vi "gwyscan create path random.vi"(5 "yoffset":dbl, 6 "xoffset":dbl, 7 "yreal":dbl, 8 "error in (no error)":errorcluster, 9 "xreal":dbl, 10 "n":i32, 11 "xypos":dbl[](array[numeric])) -> (0 "error out":errorcluster, 2 "function return":i32, 3 "xypos":dbl[](array[numeric]))   [LabVIEW 2016, in "libgwyscan.lvlib"]
doc: "GWYSCANDLL_API int gwyscan_create_path_random(double *xypos, int n, double xreal, double yreal, double xoffset, double yoffset);"
uses:
  libgwyscan.lvlib
  libgwyscan.dll
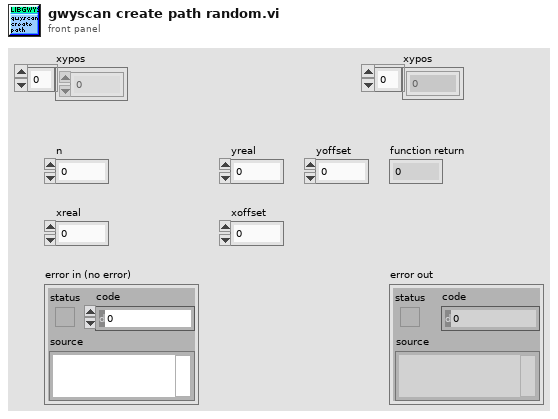
[diagram p1: front panel]
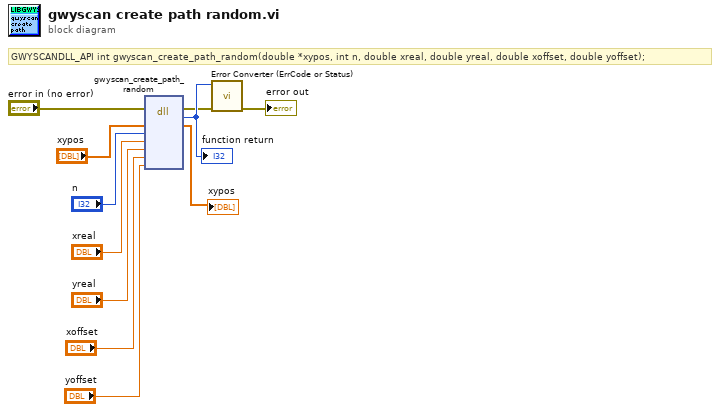
[diagram p0: block diagram]
diagram:
  # "GWYSCANDLL_API int gwyscan_create_path_random(double *xypos, int n, double xreal, double yreal, double xoffset, double yoffset);"
  n1 = dll-call lib="PTH2abs CUsersCharlÃ¨ne BrillardDesktoplbni-lbniAFMController-BetaVersionv2.0.16-20190611 libgwyscan-1.2-labview2015-win32libgwyscan.*" fn="gwyscan_create_path_random"(error in="error in (no error)", "xypos"="xypos", "n"="n", "xreal"="xreal", "yreal"="yreal", "xoffset"="xoffset", "yoffset"="yoffset") -> (error out=w3:errorcluster, "return type"=w11:i32, "xypos"=→"xypos":dbl[])  [unwired: 7 in, 1 out]
  "function return" <- w11
  n2 = call "Error Converter (ErrCode or Status).vi"("error in (no error)"=w3, "error code"=w11) -> ("error out"=→"error out":errorcluster)  [unwired: 9 in]
